vi "Panel VI Factory.vi"(6 "SubPanel?(False)":bool, 8 "error in (no error)":errorcluster, 9 "Open?(True)":bool=TRUE, 11 "Panel Control_Ref in":refnum<class "Panel Controller.lvclass">) -> (0 "error out":errorcluster, 3 "Panel Control_Ref out":refnum<class "Panel Controller.lvclass">)   [LabVIEW 2015, in "Panel Controller.lvclass"]
uses:
  Panel Controller.lvclass
panel:
  out "*(type *) &x":u16
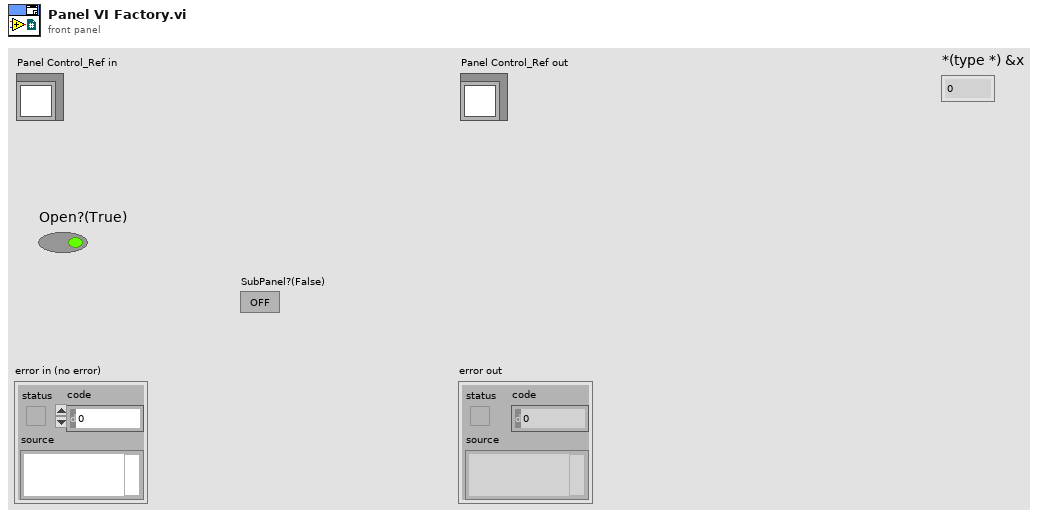
[diagram p1: front panel]
types:
  T1 = typedef "Panel Controller.lvclass/ObjectAttributes.ctl" = cluster{"Sub Panel Ref":refnum<vi>, "Panel_Q":refnum<queue>, "VI Running Refnum":refnum<vi>, "Brower Controller_Q":refnum<class "Message Enqueuer.lvclass">, "GUI Control Builder Director.lvclass":refnum<class "GUI Control Builder Director.lvclass">, "Panel GUI Manager.lvclass":refnum<class "Panel GUI Manager.lvclass">}
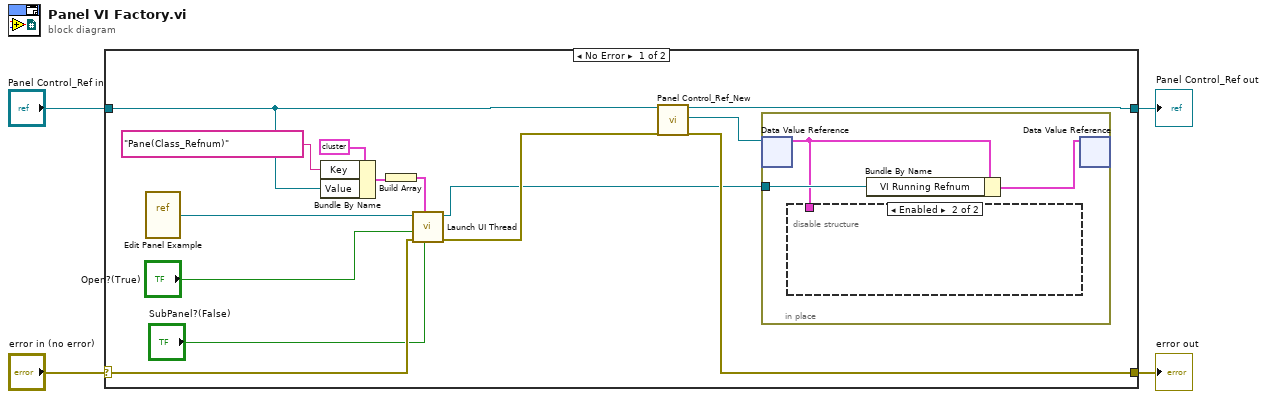
[diagram p0: block diagram]
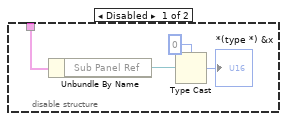
[diagram p2: hidden frame]
diagram:
  n1 = case shown="No Error" "error in (no error)" {
    selector: "error in (no error)" -> [w6 w27]
    tunnel: [w17 w27] -> w3
    tunnel: [w16 w26] -> w1
    tunnel: "Panel Control_Ref in" -> [w7 w26]
    frame No Error {
      n2 = vi-ref "Edit Panel Example.vi"() -> (w15:refnum<vi>)
      n3 = Bundle By Name(cluster=cluster{"Value":variant, "Key":string} {"Value"=variant, "Key"=""}, "Key"="Pane(Class_Refnum)", "Value"=w7) -> (w12:cluster{"Value":variant, "Key":string})
      n4 = Build Array(w12) -> (w11:cluster{"Value":variant, "Key":string}[])
      n5 = call "Launch UI Thread.vi"("SubPanel?(False)"="SubPanel?(False)", "VI Extern Value"=w11, "error in (no error)"=w6, "Open?(True)"="Open?(True)", "This VI"=w15) -> ("error out"=w9:errorcluster, "VI Running Refnum"=w8:refnum<vi>)  [unwired: 5 in]
      n6 = call "Panel Control_Ref_New.vi"("reference in"=w7, "error in (no error)"=w9) -> ("reference out"=w16:refnum<class "Panel Controller.lvclass">, "DVRRefOut"=w18:refnum<data-value>, "error out"=w17:errorcluster)  [unwired: 14 in, 1 out]
      n7 = in-place {
        in-place-border: w8 -> [w20]
        n8 = in-place-dvr #1(w18) -> (w19:T1)  [unwired: 1 out]
        n9 = disable-structure shown="Enabled" {
          disable-tunnel: w19 -> [w25 _]
          frame Disabled {
            n10 = Unbundle By Name(w25) -> ("Sub Panel Ref"=w24:refnum<vi>)
            n11 = Type Cast(type=u16 0, x=w24) -> (*(type *) &x=→"*(type *) &x":u16)
          }
          frame Enabled {
          }
        }
        n12 = Bundle By Name(cluster=w19, "VI Running Refnum"=w20) -> (w21:T1)
        n13 = in-place-dvr #1(w21) -> ()  [unwired: 2 out]
      }
    }
    frame Error {
    }
  }
  "error out" <- w3
  "Panel Control_Ref out" <- w1
